vi "RLCar_serial-tester_v1.vi"() -> ()   [LabVIEW 2021]
uses:
  <vilib>/Instr/_visa.llb/VISA Configure Serial Port (Instr).vi
  Log/_common_log/logfile-name.vi
panel:
  out "log path":string
  out "Status":string
  out "pos int":i32
  out "speed":dbl(graph)
  out "pos str":string
  in  "stop":bool
  out "Meter":dbl(knob)=26.0 scale=0.0..40.0
  out "read buffer 2":string
  out "Recovery":i32=77
  out "error out":errorcluster={"status"=FALSE, "code"=-1073807343, "source"=""}
  in  "msg":string="RLCar kit "
  in  "Led":bool
  out "seriai R feedback":i32(graph)
  in  "M dir":bool
  in  "steer":u8(slide)=26 scale=0.0..45.0
  in  "dt":u32=50
  out "read buffer":string
  out "N":i32=76
  out "seriai buff":u32(graph)
  in  "speed":u8(slide) scale=0.0..255.0
  in  "Write":bool=TRUE
  in  "rate":u32=115200
  out "String":string
  out "write buffer":string
  in  "port":refnum<visa-resource-name>="COM31"
  # "RLCar KIT control"
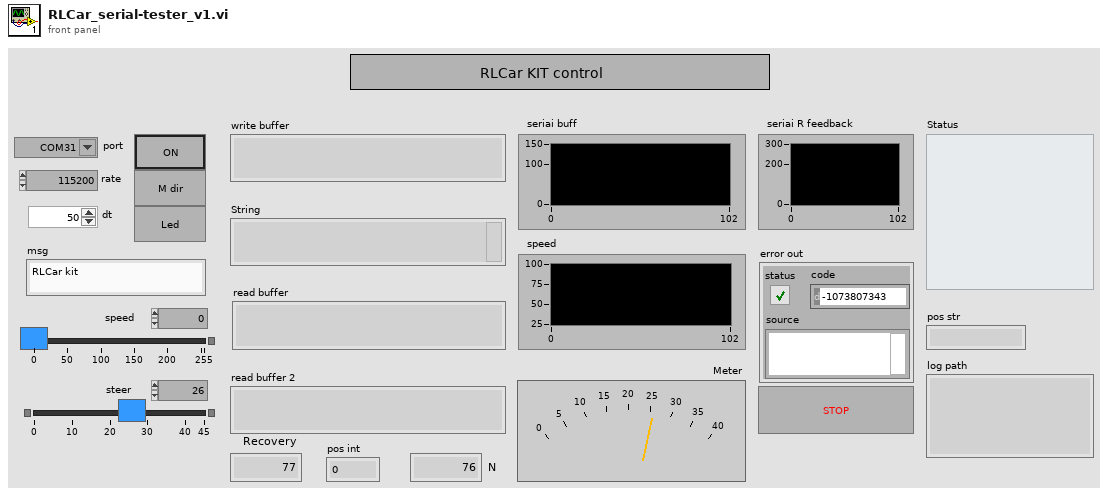
[diagram p1: front panel]
types:
  T1 = enum8{"Enabled", "Disabled", "Disabled and Grayed Out"}
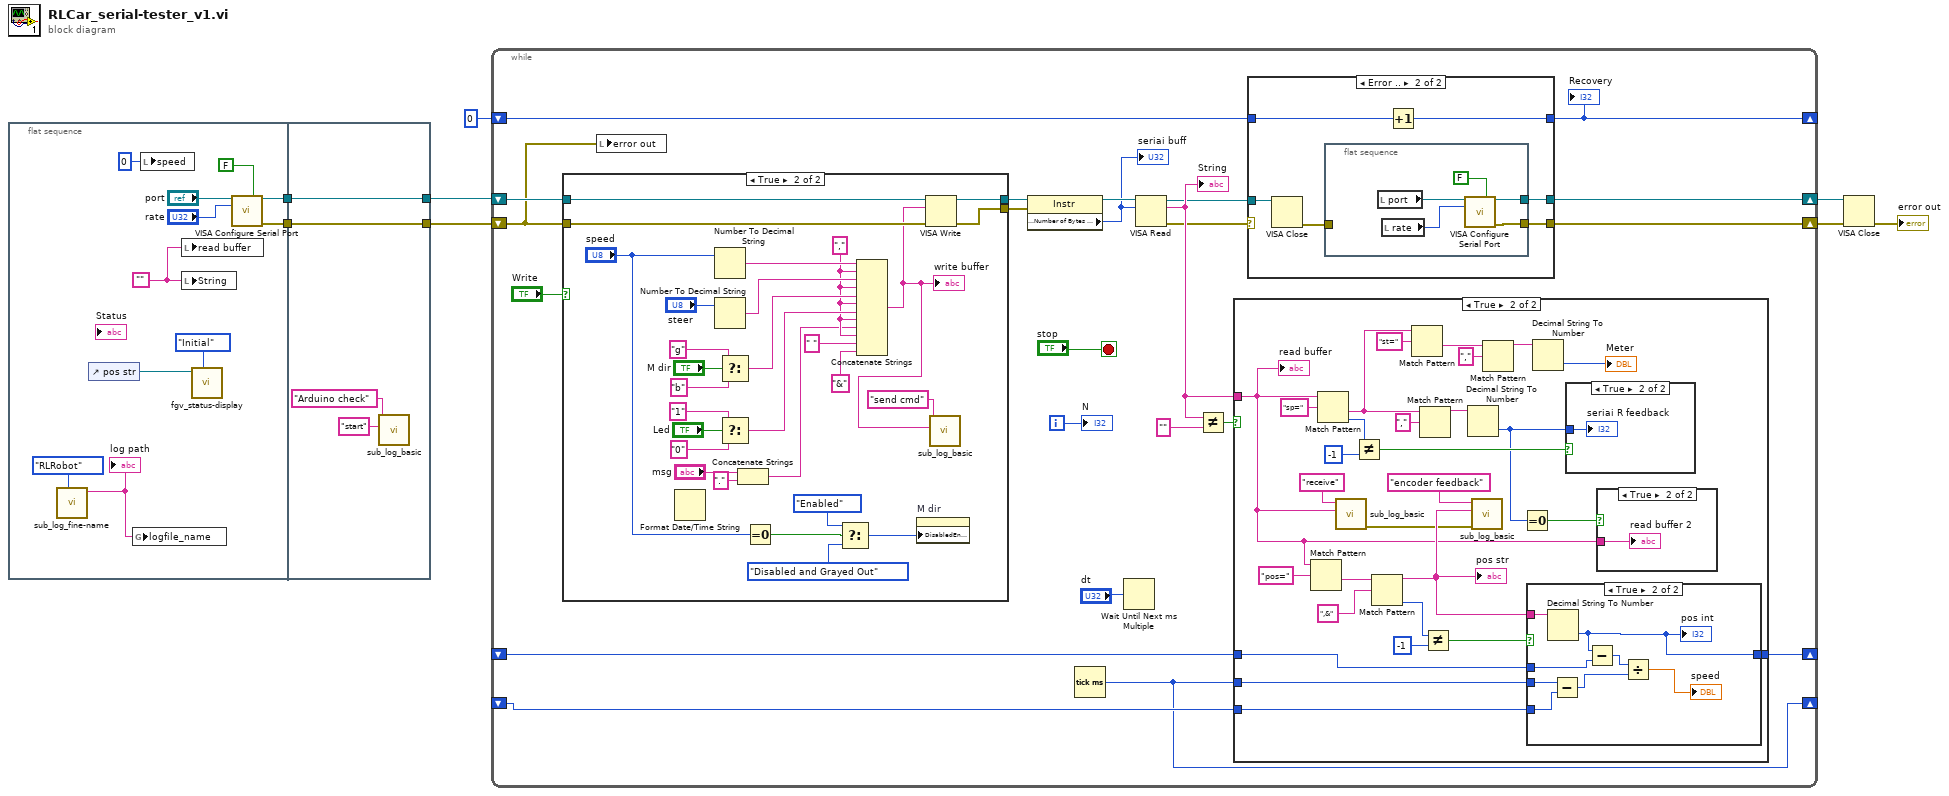
[diagram p0: block diagram]
diagram:
  n1 = flat-sequence {
    tunnel: [w18] -> w2
    tunnel: [w17] -> w1
    tunnel: [w22] -> w5
    tunnel: [w23] -> w8
    tunnel: w2 -> [w23]
    tunnel: w1 -> [w22]
    frame #0 {
      w14 = ""
      n2 = call "sub_log_fine-name.vi"("Sel"=enum16{"RLRobot", "RLGPS"}."RLRobot") -> ("log path"=w9:string)  [unwired: 10 in]
      "log path" <- w9
      n3 = control-ref of="pos str"() -> (w11:refnum<vi>)
      n4 = global write "logfile-name.vi" "logfile_name"(w9) -> ()
      n5 = local write "speed"(u8 0 ("speed")) -> ()
      n6 = local write "read buffer"(w14) -> ()
      n7 = local write "String"(w14) -> ()
      n8 = call "fgv_status-display.vi"("Mode"=enum16{"Initial", "Update", "Clear"}."Initial", "System Log"=w11) -> ()  [unwired: 9 in, 1 out]
      n9 = call-poly "VISA Configure Serial Port"("port"="port", "Enable Termination\nChar (T)"=FALSE ("Enable Termination\nChar (T)"), "baud rate (9600)"="rate") -> ("port out"=w18:refnum<visa-resource-name>, "error out"=w17:errorcluster)  [unwired: 11 in]
    }
    frame #1 {
      n10 = call "sub_log_basic.vi"("desc"="start", "Title"="Arduino check") -> ()  [unwired: 9 in, 1 out]
    }
  }
  n11 = while {
    shift-right: [w32] -> w7
    shift-left: w8 -> [w46]
    shift-right: [w33] -> w6
    shift-left: w5 -> [w29]
    shift-right: [w30] -> _
    shift-left: 0 -> [w31]
    shift-right: [w26] -> _
    shift-left: _ -> [w27]
    shift-right: [w25] -> _
    shift-left: _ -> [w24]
    i -> [w40]
    stop <- "stop" stop-if-true
    n12 = case shown="True" "Write" {
      tunnel: w46 -> [w103 w131]
      tunnel: [w102 w130] -> w41
      tunnel: w29 -> [w102 w129]
      tunnel: [w103 w128] -> w43
      frame False {
      }
      frame True {
        w115 = "," ("string")
        n13 = Format Date/Time String() -> ()  [unwired: 3 in, 1 out]
        n14 = Number To Decimal String(number="speed") -> (decimal integer string=w127:string)  [unwired: 1 in]
        n15 = Number To Decimal String(number="steer") -> (decimal integer string=w124:string)  [unwired: 1 in]
        n16 = Select(t="g" ("string"), s="M dir", f="b" ("string")) -> (s? t:f=w120:string)
        n17 = Select(t="1" ("string"), s="Led", f="0" ("string")) -> (s? t:f=w116:string)
        n18 = Concatenate Strings("msg", "." ("string")) -> (w112:string)
        n19 = Equal To 0?(x="speed") -> (x = 0?=w109:bool)
        n20 = Select(t=T1."Enabled" ("Disabled"), s=w109, f=T1."Disabled and Grayed Out" ("Disabled")) -> (s? t:f=w108:T1)
        n21 = Concatenate Strings(w127, w115, w124, w115, w120, w115, w116, w115, w112, w115, " " ("문자열"), "&" ("string")) -> (w104:string)
        "write buffer" <- w104
        n22 = property on="M dir" class="Bool (strict)"("DisabledEnum"=w108) -> ()  [unwired: 2 in, 2 out]
        n23 = VISA Write(VISA resource name=w131, write buffer=w104, error in (no error)=w129) -> (VISA resource name out=w128:refnum<visa-resource-name>, error out=w130:errorcluster)  [unwired: 1 out]
        n24 = call "sub_log_basic.vi"("desc"=w104, "Title"="send cmd") -> ()  [unwired: 9 in, 1 out]
      }
    }
    n25 = local write "error out"(w29) -> ()
    n26 = property class="Instr"(reference=w43, error in=w41) -> (reference out=w44:refnum<visa-resource-name>, "Serial Settings:Number of Bytes at Serial Port"=w39:u32)  [unwired: 1 out]
    "seriai buff" <- w39
    n27 = Tick Count (ms)() -> (millisecond timer value=w26:u32)
    n28 = Wait Until Next ms Multiple(millisecond multiple="dt") -> ()  [unwired: 1 out]
    n29 = VISA Read(VISA resource name=w44, byte count=w39) -> (VISA resource name out=w34:refnum<visa-resource-name>, read buffer=w36:string, error out=w35:errorcluster)  [unwired: 1 in, 1 out]
    "String" <- w36
    n30 = Not Equal?(x=w36, y="") -> (x != y?=w37:bool)
    n31 = case shown="True" w37 {
      tunnel: w36 -> [_ w63]
      tunnel: w27 -> [_ w70]
      tunnel: w26 -> [_ w69]
      tunnel: [w61 w68] -> w25
      tunnel: w24 -> [w61 w67]
      frame False {
      }
      frame True {
        n32 = Match Pattern(string=w63, regular expression="pos=" ("정규식")) -> (after substring=w74:string)  [unwired: 1 in, 3 out]
        n33 = Match Pattern(string=w63, regular expression="sp=" ("정규식")) -> (after substring=w84:string, offset past match=w81:i32)  [unwired: 1 in, 2 out]
        n34 = call "sub_log_basic.vi"("desc"=w63, "Title"="receive") -> ("error out"=w62:errorcluster)  [unwired: 9 in]
        n35 = Not Equal?(x=w81, y=-1) -> (x != y?=w79:bool)
        n36 = Match Pattern(string=w74, regular expression=",&") -> (before substring=w65:string, offset past match=w72:i32)  [unwired: 1 in, 2 out]
        "pos str" <- w65
        n37 = Match Pattern(string=w84, regular expression="st=" ("정규식")) -> (after substring=w83:string)  [unwired: 1 in, 3 out]
        n38 = Match Pattern(string=w84, regular expression="," ("정규식")) -> (before substring=w88:string)  [unwired: 1 in, 3 out]
        n39 = Not Equal?(x=w72, y=-1) -> (x != y?=w71:bool)
        n40 = Decimal String To Number(string=w88) -> (number=w78:i32)  [unwired: 2 in, 1 out]
        n41 = call "sub_log_basic.vi"("error in"=w62, "desc"=w65, "Title"="encoder feedback") -> ()  [unwired: 8 in, 1 out]
        n42 = Match Pattern(string=w83, regular expression="," ("정규식")) -> (before substring=w87:string)  [unwired: 1 in, 3 out]
        n43 = Equal To 0?(x=w78) -> (x = 0?=w82:bool)
        n44 = case shown="True" w71 {
          tunnel: w65 -> [_ w99]
          tunnel: w70 -> [_ w97]
          tunnel: w69 -> [_ w98]
          tunnel: [w91 w94] -> w68
          tunnel: w67 -> [w91 w93]
          frame False {
          }
          frame True {
            n45 = Decimal String To Number(string=w99) -> (number=w94:i32)  [unwired: 2 in, 1 out]
            "pos int" <- w94
            n46 = Subtract(x=w98, y=w97) -> (x-y=w96:u32)
            n47 = Subtract(x=w94, y=w93) -> (x-y=w92:i32)
            n48 = Divide(x=w92, y=w96) -> (x/y=→"speed":dbl)
          }
        }
        n49 = Decimal String To Number(string=w87) -> (number=→"Meter":i32)  [unwired: 2 in, 1 out]
        n50 = case shown="True" w79 {
          tunnel: w78 -> [_ w100]
          frame False {
          }
          frame True {
            "seriai R feedback" <- w100
          }
        }
        n51 = case shown="True" w82 {
          tunnel: w63 -> [_ w101]
          frame False {
          }
          frame True {
            "read buffer 2" <- w101
          }
        }
        "read buffer" <- w63
      }
    }
    n52 = case shown="Error .." w35 {
      selector: w35 -> [w48 _]
      tunnel: w34 -> [w49 w55]
      tunnel: [w48 w53] -> w33
      tunnel: [w49 w52] -> w32
      tunnel: w31 -> [w47 w51]
      tunnel: [w47 w50] -> w30
      frame No Error {
      }
      frame Error {
        n53 = VISA Close(VISA resource name=w55) -> (error out=w54:errorcluster)  [unwired: 1 in]
        n54 = flat-sequence {
          tunnel: w54 -> [_]
          tunnel: [w57] -> w53
          tunnel: [w56] -> w52
          frame #0 {
            n55 = local read "port"() -> (w59:refnum<visa-resource-name>)
            n56 = local read "rate"() -> (w58:u32)
            n57 = call-poly "VISA Configure Serial Port"("port"=w59, "Enable Termination\nChar (T)"=FALSE ("Enable Termination\nChar (T)"), "baud rate (9600)"=w58) -> ("port out"=w56:refnum<visa-resource-name>, "error out"=w57:errorcluster)  [unwired: 11 in]
          }
        }
        n58 = Increment(x=w51) -> (x+1=w50:i32)
      }
    }
    "Recovery" <- w30
    "N" <- w40
  }
  n59 = VISA Close(VISA resource name=w7, error in (no error)=w6) -> (error out=→"error out":errorcluster)
